vi "Pre Launch Init.vi"(11 "Nested in":refnum<class "UI_Top_Customer.lvclass">) -> (0 "error out":errorcluster, 3 "Nested out":refnum<class "UI_Top_Customer.lvclass">)   [LabVIEW 2021, in "UI_Top_Customer.lvclass"]
doc: "(<B>Filename</B>: Actor Framework.lvlib:Actor.lvclass:Pre Launch Init.vi)\n\nDefines behavior that occurs after the Launch Nested Actor method is invoked but before the actor's Actor Core method begins running.\n\nBy default, this method does nothing. A descendant class may override it to define behavior."
uses:
  UI_Top_Customer.lvclass
  UI_Top_Customer.lvclass/UI_Top_Customer.ctl
  <userlib>/John_Lib/AbstractActorTemplate/AbstractActorTemplate/UIActorTop.lvclass
  <userlib>/John_Lib/Queue_Self/Queue_Self.lvlib
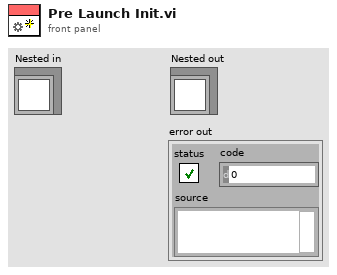
[diagram p1: front panel]
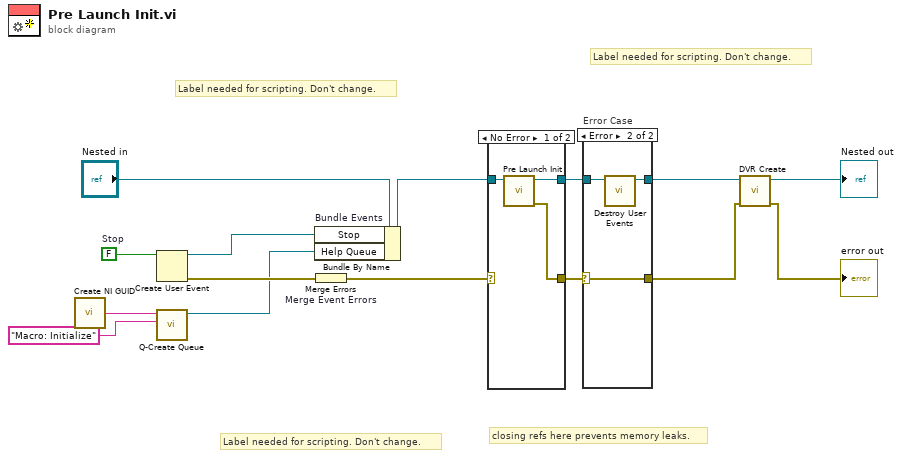
[diagram p0: block diagram]
diagram:
  w14 = FALSE  # Stop
  # "Label needed for scripting. Don't change."
  # "Label needed for scripting. Don't change."
  # "Label needed for scripting. Don't change."
  # "closing refs here prevents memory leaks."
  n1 = call <vilib>:"Create NI GUID.vi"() -> ("NI GUID"=w3:string)
  n2 = Create User Event(user event datatype=w14) -> (user event=w12:refnum<user-event>, error out=w13:errorcluster)  [unwired: 1 in]
  n3 = call <userlib>:"Q-Create Queue.vi"("CMD"="Macro: Initialize" ("initial message names"), "message queue name"=w3) -> ("queue out"=w1:refnum<queue>)  [unwired: 8 in, 1 out]
  n4 = Bundle By Name "Bundle Events"(cluster="Nested in", "Stop"=w12, "Help Queue"=w1) -> (w10:refnum<class "UI_Top_Customer.lvclass">)
  n5 = Merge Errors "Merge Event Errors"(w13) -> (w9:errorcluster)
  n6 = case shown="No Error" w9 {
    selector: w9 -> [_ w20]
    tunnel: [w18 w19] -> w11
    tunnel: w10 -> [w17 w19]
    tunnel: [w16 w20] -> w8
    frame No Error {
      n7 = call-parent "Pre Launch Init.vi"("Actor in"=w17) -> ("error out"=w16:errorcluster, "Actor out"=w18:refnum<class "UI_Top_Customer.lvclass">)  [unwired: 9 in]
    }
    frame Error {
    }
  }
  n8 = case "Error Case" shown="Error" w8 {
    selector: w8 -> [w21 w25]
    tunnel: w11 -> [w22 w24]
    tunnel: [w22 w23] -> w7
    tunnel: [w21 w25] -> w5
    frame No Error {
    }
    frame Error {
      n9 = call "Destroy User Events.vi"("UI Template in"=w24) -> ("UI Template out"=w23:refnum<class "UI_Top_Customer.lvclass">)  [unwired: 10 in]
    }
  }
  n10 = call "DVR Create.vi"("error in (no error)"=w5, "UI_Top_Customer in"=w7) -> ("error out"=→"error out":errorcluster, "UI_Top_Customer out"=→"Nested out":refnum<class "UI_Top_Customer.lvclass">)  [unwired: 8 in]
